vi "GetStatus.vi"(8 "error in (no error)":errorcluster, 11 "AODAcq in":refnum<class "AODAcq.lvclass">) -> (0 "error out":errorcluster, 2 "Status":T2, 3 "AODAcq out":refnum<class "AODAcq.lvclass">)   [LabVIEW 2014, in "AODAcq.lvclass"]
uses:
  AODAcq.lvclass
  FPGA_Control/FPGAState.ctl
  <vilib>/Utility/error.llb/Error Cluster From Error Code.vi
  C:/Program Files (x86)/National Instruments/LabVIEW 2014/Targets/NI/FPGA/StockFPGA_IntfPrivate/ScriptTemplates/StockFPGA_PlugInRead32.vi
  <vilib>/rvi/errors/niLvFpgaAdjustHostInterfaceError.vi
  <vilib>/rvi/interface/nirviReadWriteControl/nirviReadWriteControl.xnode
  FPGA_Control/AODRef.ctl
  FPGA Bitfiles/AodScanner_FPGATarget_AODControl(FPGA)_TyJc9yYmyGA.lvbitx
  NiFpgaLv.dll
  <vilib>/FPGAPlugInAG/PXIe-7965R/niLvFpga_Read32_PXIe-7965R.vi
  <vilib>/rvi/interface/nirviReadWriteControl/niFpgaRWControlAccessTimeoutTemplate.vi
panel:
  out "Error.Sequencer":bool
  out "Error.Serial error":bool
  out "Error.UpdateIOTimeout":bool
  out "Error.OutOfRange":bool
  out "Status.Sequencer":T1
  out "Status.AcqState":enum16{"Idling", "Acquiring"}(ring)
  out "Status.Last Point":bool
  out "Scan.Acquire Samples":u32
  in  "index":i32
  out "Waveform Chart":i16(graph)
  out "Analog Data":i16[](array[numeric])
  out "Status.All Samples":bool
  out "Status.Update IO Missing":bool
  out "Status.TemporalChFull":bool
  out "Scan.NumPoints":u32
  out "Status.DownsampleDone":bool
  out "Status.MotionChFull":bool
  out "Status.ImChFull":bool
  out "Scan.NumMotionPoints":u32
  out "Scan.Motion Increment":u32
  out "Scan.TotalSamples":u32
  out "Debug.PMT_Unpacked_backlog":u32
  out "Debug.PMT_Data_backlog":u32
  out "Comm.CommLines":enum16{"1", "2", "4"}(ring)
  out "Comm.WriteCount":i32
  out "Comm.Written":cluster{"Address":u8, "Value":u32}[](array[cluster])
  out "Debug.Point":cluster{"X":i32, "Y":i32, "Z":i32}
  out "Status.BufferedPoints":i32
  out "Debug.PMT_Samples":u32
  out "Scan.Samples":u32
  out "Debug.PMT Array":i32[](array[numeric])
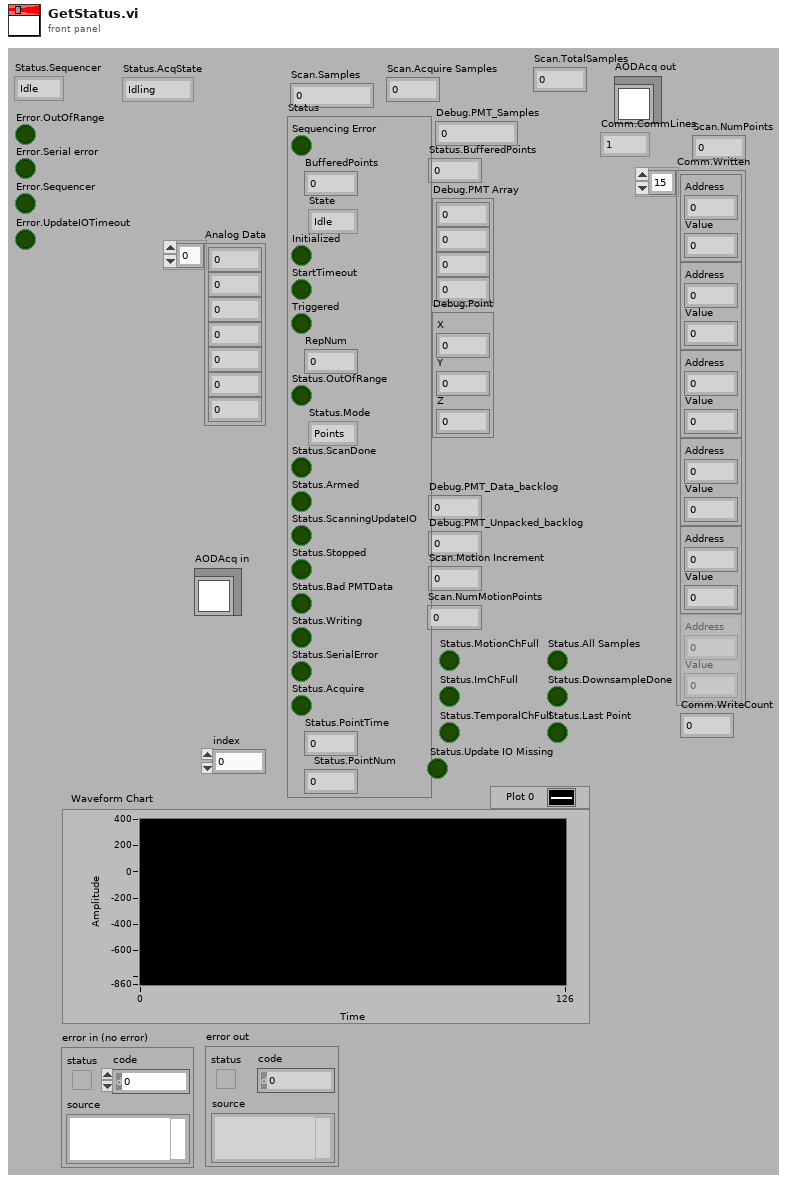
[diagram p1: front panel]
types:
  T1 = typedef "FPGAState.ctl" = enum16{"Idle", "Arm Scan", "Scan", "End Scan"}
  T2 = cluster{"Sequencing Error":bool, "BufferedPoints":i32, "State":T1, "Initialized":bool, "StartTimeout":bool, "Triggered":bool, "RepNum":u32, "Status.OutOfRange":bool, "Status.Mode":enum16{"Points", "Volume", "Idle"}, "Status.ScanDone":bool, "Status.Armed":bool, "Status.ScanningUpdateIO":bool, "Status.Stopped":bool, "Status.Bad PMTData":bool, "Status.Writing":bool, "Status.SerialError":bool, "Status.Acquire":bool, "Status.PointTime":u32, "Status.PointNum":u64}
  T3 = typedef "AODRef.ctl" = refnum<k20>
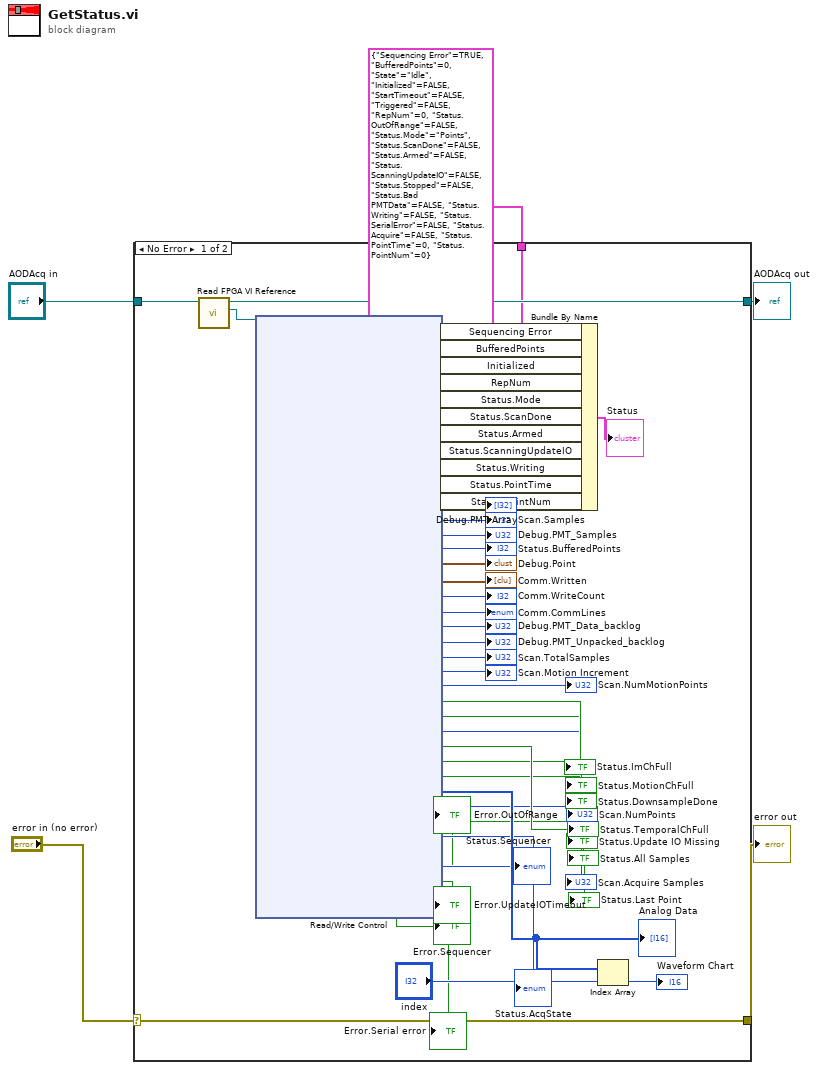
[diagram p0: block diagram]
diagram:
  n1 = case shown="No Error" "error in (no error)" {
    selector: "error in (no error)" -> [w52 w54]
    tunnel: [w52 w54] -> w4
    tunnel: [w50 w53] -> w2
    tunnel: "AODAcq in" -> [w51 w53]
    tunnel: T2 {"Sequencing Error"=TRUE, "BufferedPoints"=0, "State"=enum."Idle", "Initialized"=FALSE, "StartTimeout"=FALSE, "Triggered"=FALSE, "RepNum"=0, "Status.OutOfRange"=FALSE, "Status.Mode"=enum."Points", "Status.ScanDone"=FALSE, "Status.Armed"=FALSE, "Status.ScanningUpdateIO"=FALSE, "Status.Stopped"=FALSE, "Status.Bad PMTData"=FALSE, "Status.Writing"=FALSE, "Status.SerialError"=FALSE, "Status.Acquire"=FALSE, "Status.PointTime"=0, "Status.PointNum"=0} -> [w46 _]
    frame No Error {
      n2 = call-dynamic "Read FPGA VI Reference.vi"("AODAcq in"=w51) -> ("FPGA VI Reference"=w49:T3, "AODAcq out"=w50:refnum<class "AODAcq.lvclass">)  [unwired: 8 in, 1 out]
      n3 = xnode "Read/Write Control"("FPGA VI Reference In"=w49) -> ("Status.Sequencing error"=w48:bool, "Status.BufferedPoints"=w47:i32, "Status.Initialized"=w45:bool, "Status.RepNum"=w44:u32, "Status.Mode"=w43:enum16{"Points", "Volume", "Idle"}, "Status.ScanDone"=w42:bool, "Status.Armed"=w41:bool, "Status.ScanUpdateIO"=w40:bool, "Status.Writing"=w37:bool, "Status.PointTime"=w38:u32, "Status.PointNum"=w39:u32, "Debug.PMT Array"=→"Debug.PMT Array":i32[], "Scan.SampleToLoad"=→"Scan.Samples":u32, "Debug.PMT_Samples"=→"Debug.PMT_Samples":u32, "Status.BufferedPoints"=→"Status.BufferedPoints":i32, "Debug.Point"=→"Debug.Point":cluster{"X":i32, "Y":i32, "Z":i32}, "Comm.Write"=→"Comm.Written":cluster{"Address":u8, "Value":u32}[], "Comm.WritenCount"=→"Comm.WriteCount":i32, "Comm.CommLines"=→"Comm.CommLines":enum16{"1", "2", "4"}, "Debug.PMT_Data_backlog"=→"Debug.PMT_Data_backlog":u32, "Debug.PMT_Unpacked_backlog"=→"Debug.PMT_Unpacked_backlog":u32, "Scan.TotalSamples"=→"Scan.TotalSamples":u32, "Scan.Motion Increment"=→"Scan.Motion Increment":u32, "Scan.NumMotionPoints"=→"Scan.NumMotionPoints":u32, "Status.ImChFull"=→"Status.ImChFull":bool, "Status.MotionChFull"=→"Status.MotionChFull":bool, "Scan.NumPoints"=→"Scan.NumPoints":u32, "Status.TemporalChFull"=→"Status.TemporalChFull":bool, "Status.Update IO Missing"=→"Status.Update IO Missing":bool, "Status.All Samples"=→"Status.All Samples":bool, "Analog Data"=w15:i16[], "Scan.Acquire Samples"=→"Scan.Acquire Samples":u32, "Status.Last Point"=→"Status.Last Point":bool, "Status.AcqState"=→"Status.AcqState":enum16{"Idling", "Acquiring"}, "Status.Sequencer"=→"Status.Sequencer":T1, "Error.OutOfRange"=→"Error.OutOfRange":bool, "Error.UpdateIOTimeout"=→"Error.UpdateIOTimeout":bool, "Error.Serial error"=→"Error.Serial error":bool, "Error.Sequencer"=→"Error.Sequencer":bool)  [unwired: 1 in, 2 out]
      "Analog Data" <- w15
      n4 = Bundle By Name(cluster=w46, "Sequencing Error"=w48, "BufferedPoints"=w47, "Initialized"=w45, "RepNum"=w44, "Status.Mode"=w43, "Status.ScanDone"=w42, "Status.Armed"=w41, "Status.ScanningUpdateIO"=w40, "Status.Writing"=w37, "Status.PointTime"=w38, "Status.PointNum"=w39) -> (→"Status":T2)
      n5 = Index Array(array=w15, index="index") -> (element=→"Waveform Chart":i16)
    }
    frame Error {
    }
  }
  "error out" <- w4
  "AODAcq out" <- w2
